vi "Stop Core.vi"(10 "final error code":i32, 11 "Sample Error Reporter in":refnum<class "Sample Error Reporter.lvclass">) -> (3 "Sample Error Reporter out":refnum<class "Sample Error Reporter.lvclass">)   [LabVIEW 2024, in "Sample Error Reporter.lvlib" / "Sample Error Reporter.lvclass"]
doc: "<p>(<strong>Filename</strong>: <span class=\"dnl\">Actor Framework.lvlib:Actor.lvclass:Stop Core.vi</span>)</p>\n<p>Defines what the actor does before it stops. Use the <strong>final error code</strong> input to determine whether the actor shut down in response to an error.</p>\n<p>By default, this method passes the Stop message along to all <a href=\"nihelplauncher://docs/csh?context=lvcore_lvcomm_af_launch_nested_actor\">auto-stop nested actors</a>. A descendant class may override this method to define additional behavior, such as shutting down any processes the actor initiated in its override of the <a href=\"nihelplauncher://docs/csh?context=lvcore_lvcomm_af_actor_core\">Actor Core</a> method.</p>"
uses:
  Sample Error Reporter.lvclass
  Sample Error Reporter.lvclass/Sample Error Reporter.ctl
  src/Error Reporting Actor/Error Reporter/Error Reporter/Error Reporter.lvclass
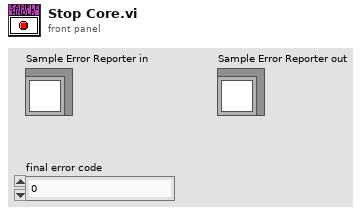
[diagram p1: front panel]
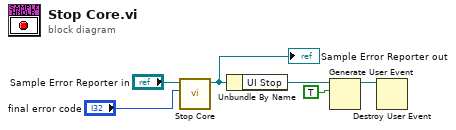
[diagram p0: block diagram]
diagram:
  n1 = call-parent "Stop Core.vi"("final error code"="final error code", "Error Reporter in"="Sample Error Reporter in") -> ("Error Reporter out"=w4:refnum<class "Sample Error Reporter.lvclass">)  [unwired: 9 in]
  "Sample Error Reporter out" <- w4
  n2 = Unbundle By Name(w4) -> ("UI Stop"=w3:refnum<user-event>)
  n3 = Generate User Event(user event=w3, event data cluster=TRUE ("event data")) -> (user event out=w2:refnum<user-event>)  [unwired: 2 in, 1 out]
  n4 = Destroy User Event(user event=w2) -> ()  [unwired: 1 in, 1 out]
